vi "Zählerwert_setzen.vi"(8 "gewünschter Zählerwert":u16, 9 "Zähler":enum16{"Zähler 1", "Zähler 2", "Zähler 3"}(ring), 11 "Band/Station Index":T1) -> ()   [LabVIEW 2013, in "cRIO_FPGA_COMMUNICATION.lvlib"]
uses:
  cRIO_FPGA_COMMUNICATION.lvlib
  TYPES/TYPE Station Index.ctl
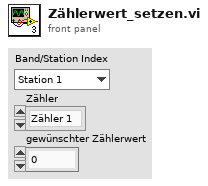
[diagram p1: front panel]
types:
  T1 = typedef "cRIO_FPGA_COMMUNICATION.lvlib/TYPE Station Index.ctl" = enum16{"Station 1", "Station 2", "Station 3", "Station 4", "Station 5", "Station 6", "Station 7", "Station 8", "Station 9", "Station 10", "Station 11", "Station 12", "Station 13", "Station 14", "Station 15", "Station 16", "Station 17", "Station 18", "Station 19", "Station 20"}
  T2 = enum16{"Init", "Zählerwert nullen", "Zählerwert setzen", "lese gesetzten Zählerwert"}
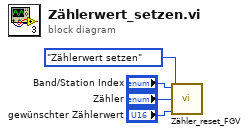
[diagram p0: block diagram]
diagram:
  n1 = call "Zähler_reset_FGV.vi"("Band/Station Index"="Band/Station Index", "Modus"=T2."Zählerwert setzen", "gewünschter Zählerwert"="gewünschter Zählerwert", "Zähler"="Zähler") -> ()  [unwired: 1 in, 3 out]
